vi "Write Param Referense.vi"(8 "error in (no error)":errorcluster, 10 "Param Referense":T1, 11 "MB_TCP in":refnum<class "MB_TCP.lvclass">) -> (0 "error out":errorcluster, 3 "MB_TCP out":refnum<class "MB_TCP.lvclass">)   [LabVIEW 2019, in "MB_TCP.lvclass"]
uses:
  MB_TCP.lvclass
  ICPCON Param/ICPCON Param.ctl
  ICPCON Param/Eth timeouts.ctl
  MB_TCP.lvclass/MB_TCP.ctl
  ICPCON Param/ICPCON_Param.lvlib
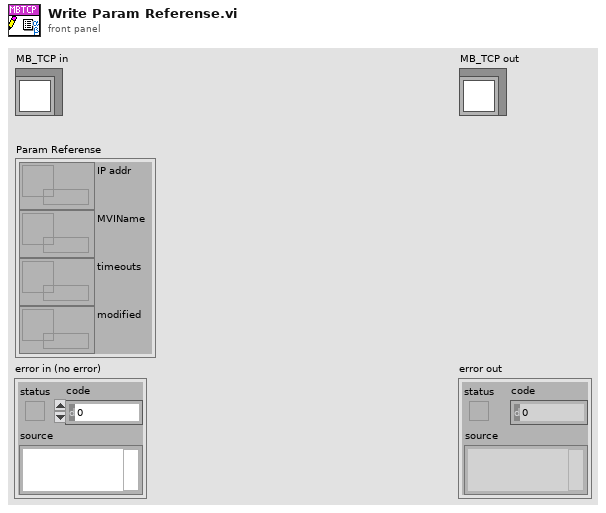
[diagram p1: front panel]
types:
  T1 = typedef "ICPCON_Param.lvlib/ICPCON Param.ctl" = cluster{"IP addr":refnum<data-value>, "MVIName":refnum<data-value>, "timeouts":refnum<data-value>, "modified":refnum<data-value>}
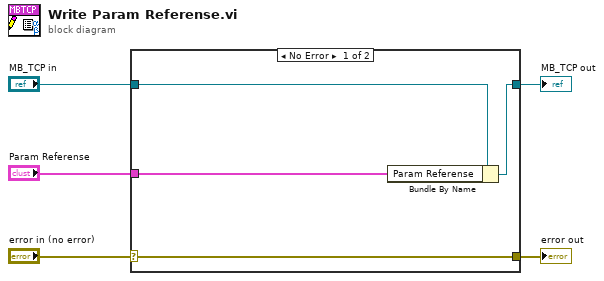
[diagram p0: block diagram]
diagram:
  n1 = case shown="No Error" "error in (no error)" {
    selector: "error in (no error)" -> [w9 w10]
    tunnel: [w9 w10] -> w4
    tunnel: [w7 w11] -> w2
    tunnel: "MB_TCP in" -> [w8 w11]
    tunnel: "Param Referense" -> [w6 _]
    frame No Error {
      n2 = Bundle By Name(cluster=w8, "Param Referense"=w6) -> (w7:refnum<class "MB_TCP.lvclass">)
    }
    frame Error {
    }
  }
  "error out" <- w4
  "MB_TCP out" <- w2
